vi "CSM - With Event Structure Template.vi"(5 "Init State(\"Macro: Initialize\")":string="Macro: Initialize", 7 "Name(\"\" to use uuid)":string="Event CSM") -> ()   [LabVIEW 2014]
doc: "Template for building CSM Module with User Interface. Event Structure is included in template for processing user operations.\n\n<b>Inputs:</b>\n - <b>Name(\"\" to use uuid)</b>: Module Name\n - If Input is \"\", an uuid will be used for module name. The module is marked as stand-alone mode and will not be included in module list.\n - Fi Input end with '#', the module will worked in worker mode. Modules with the same name will shared the same message queue. Any external message will be processed by one of the modules, depending who is free.\n - Otherwise, the input string will be used as module name, which should be unique in system. CSM will go to \"Critical Error\" state if duplicated module name is used in system.\n\n<b>Outputs:</b>\n - N/A"
uses:
  _Support/Priority Queue/Priority Queue.lvclass/Priority Queue.ctl
  AdvanceAPI/CSM - Revert Arguments-Safe String.vi
  _Support/Common/Trim Single line Text.vi
  _Support/Process/CSMP-Async Call.vi
  _Support/GlobalEvent/GEvt-Generate Status Log.vi
  _Support/Process/CSMP-Broadcast.vi
  _Support/GlobalEvent/GEvt-Generate Interrupt Log.vi
  _Support/GlobalEvent/GEvt-Generate Register Log.vi
  _Support/Process/CSMP-Register Status.vi
  _Support/GlobalEvent/GEvt-Generate Unregister Log.vi
  _Support/Process/CSMP-Unregister Status.vi
  _Support/Process/CSMP-Sync Call.vi
  _Support/CSMQ/_CSMObj-Unlock.vi
  _Support/Process/CSMP-PostPostMsg.vi
  _Support/Process/CSMP-PostSendMsg.vi
  _Support/CSMQ/_CSMObj-Lock State.vi
  _Support/Common/Splite Reason String Part.vi
  _Support/CSMQ/_CSMOFGV Release.vi
  _Support/Common/Remove Comments from Line.vi
  _Support/Common/Splite Single-line Message.vi
  _Support/Common/Parse Next Single-line State.vi
  _Support/CSMQ/_CSMOFGV Dequeue.vi
  _Support/CSMQ/_CSMObj-Log Error if in a Remote Session.vi
  _Support/GlobalEvent/GEvt-Generate State Change Log.vi
  _Support/GlobalEvent/GEvt-Generate Remaining States Log.vi
  _Support/GlobalEvent/GEvt-Generate Complete Log.vi
  AdvanceAPI/CSM - Keywords.vi
  _Support/CSMQ/_CSMObj-Message Check.vi
  _Support/CSMQ/_CSMObj-Enqueue Cross-Module Message.vi
  _Support/CSMQ/_CSMOFGV Get.vi
  _Support/FGV-BroadcastRegistry/Cache-Broadcast Registry Search Result.vi
  AdvanceAPI/CSM - Register Status Change.vi
  AdvanceAPI/CSM - Unregister Status Change.vi
  _Support/Common/Hex Str to U8 Data.vi
  _Support/Common/Concatenate State with Arguments.vi
  _Support/Common/U8 Data to Hex Str.vi
  Build State String with Arguments++.vi
  _Support/Priority Queue/Dequeue Element.vi
  _Support/Priority Queue/Enqueue Element.vi
  Utility/Trim Both Whitespace.vi
  _Support/CSMQ/_CSMOFGV.vi
  Utility/Build Error Cluster.vi
  _Support/FGV-BroadcastRegistry/FGV-BroadcastRegistry.vi
  _Support/FGV-BroadcastRegistry/global-Broadcast Cache Change Flag.vi
  _Support/GlobalEvent/FGV-StatusChangeEventRef.vi
  _Support/CSMQ/_CSMOFGV Obtain.vi
  _Support/GlobalEvent/FGV-GlobalEventRef.vi
  Communicable State Machine.lvlib
panel:
  out "State History":string
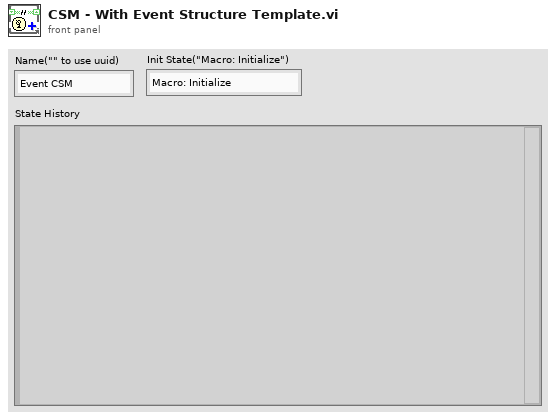
[diagram p1: front panel]
types:
  T1 = enum32{"Invalid", "Standard", "Closed", "Hidden", "Minimized", "Maximized"}
  T2 = enum32{"invalid app kind", "Development System", "Run Time System", "Student Edition", "Embedded LabVIEW", "Evaluation", "Custom"}
  T3 = typedef "Communicable State Machine.lvlib/_CSM_Response Source Message.ctl" = cluster{"‘State":string, "’Arguments":string, "’Error":errorcluster}
  T4 = cluster{"Core":cluster{"Current VI Reference":refnum<vi>, "Close Panel on Exit?":bool}, "Your Boolean data":bool, "Your string data":string}
  T5 = cluster{"Current VI Reference":refnum<vi>, "Close Panel on Exit?":bool}
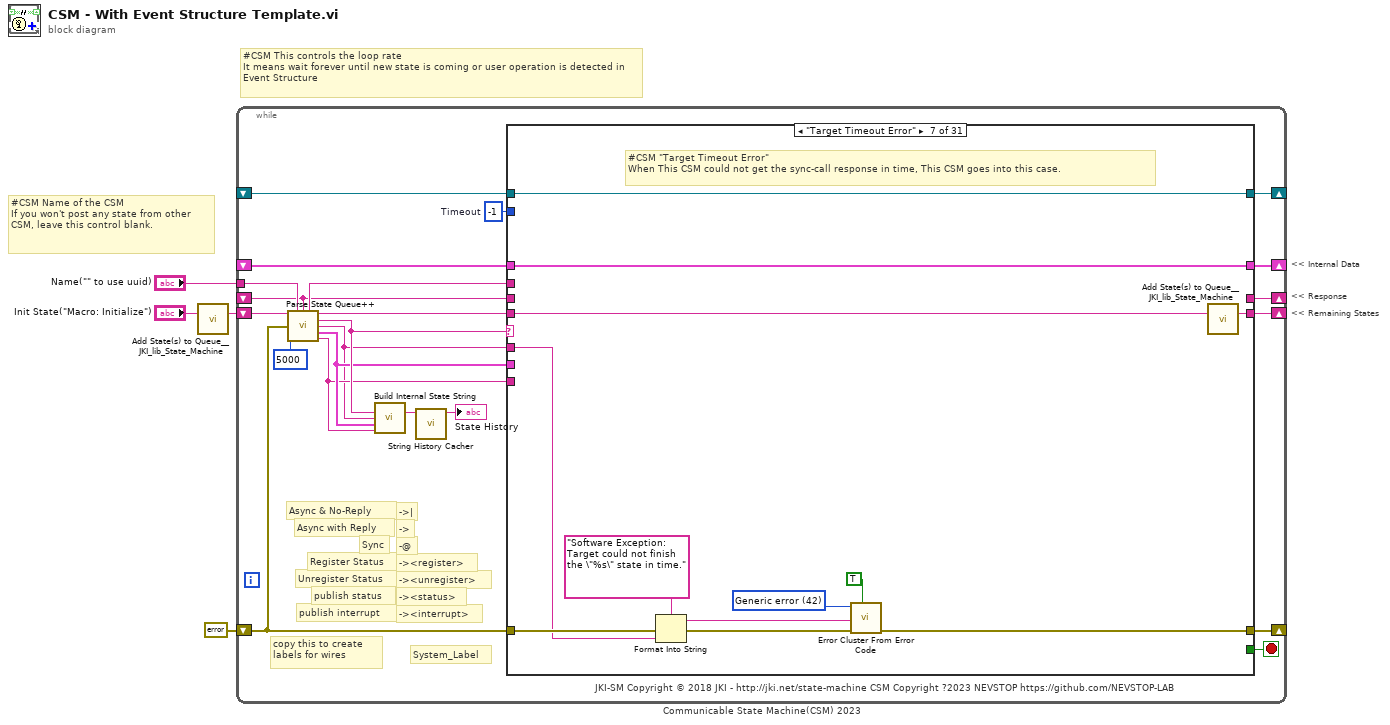
[diagram p0: block diagram]
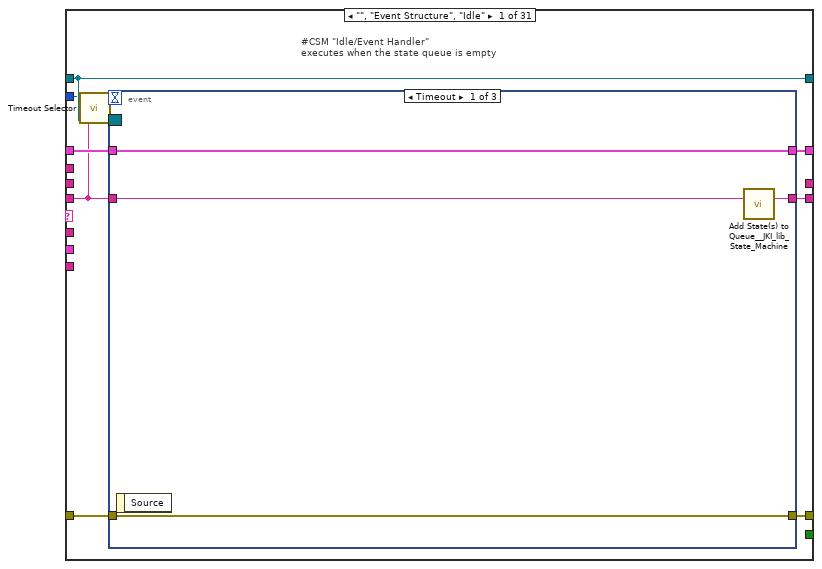
[diagram p2: hidden frame]
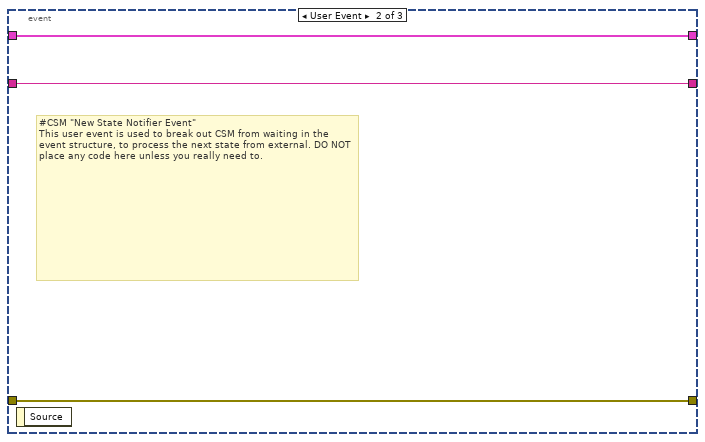
[diagram p3: hidden frame]
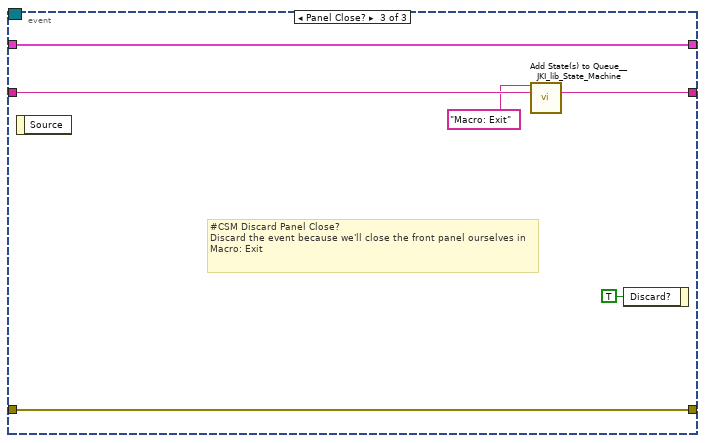
[diagram p4: hidden frame]
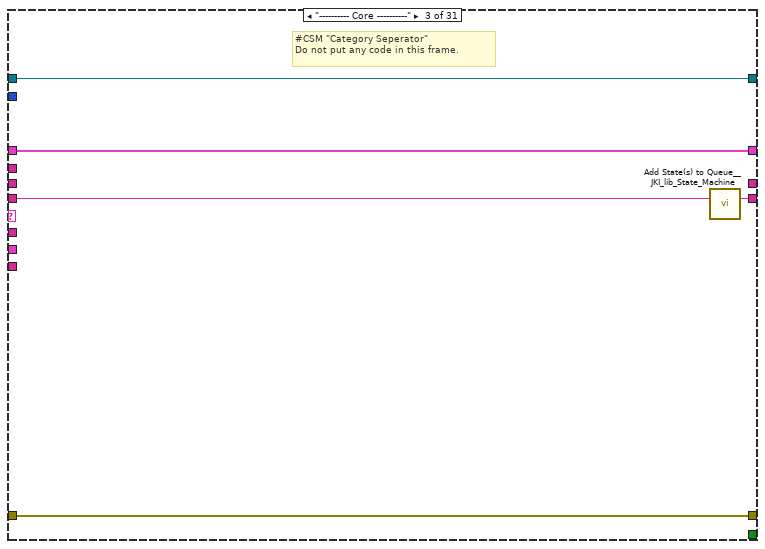
[diagram p6: hidden frame]
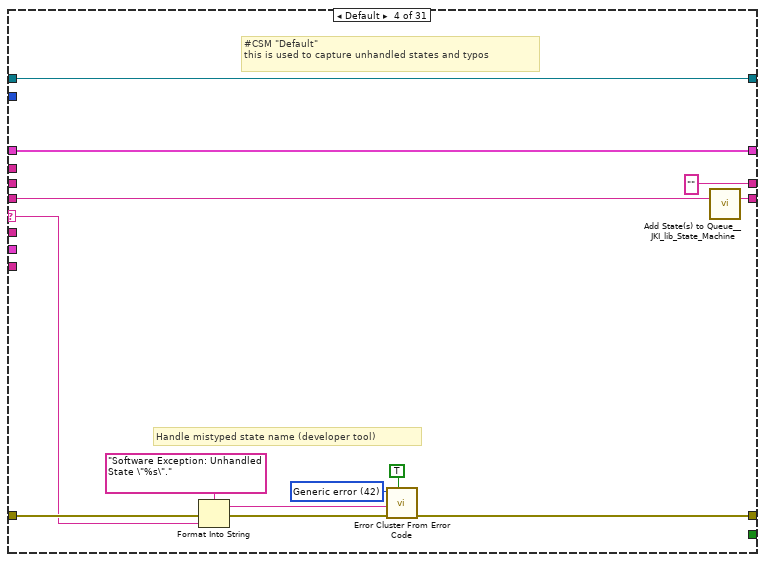
[diagram p7: hidden frame]
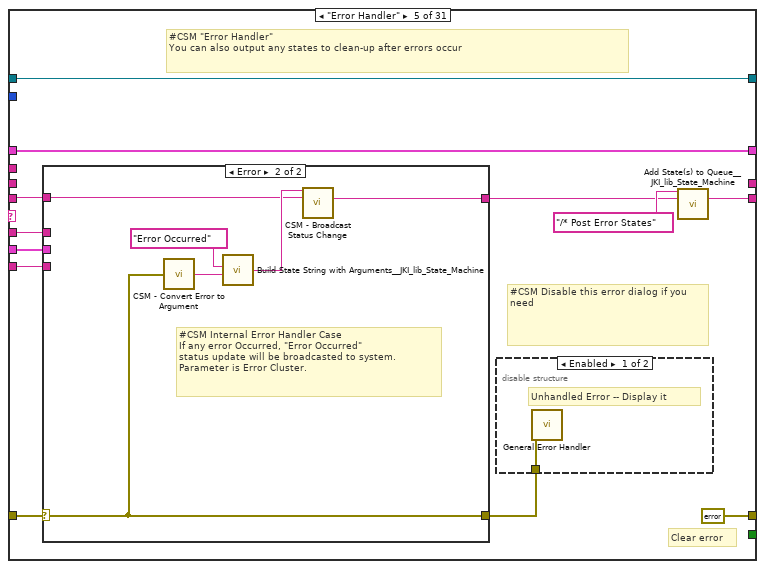
[diagram p8: hidden frame]
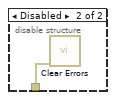
[diagram p9: hidden frame]
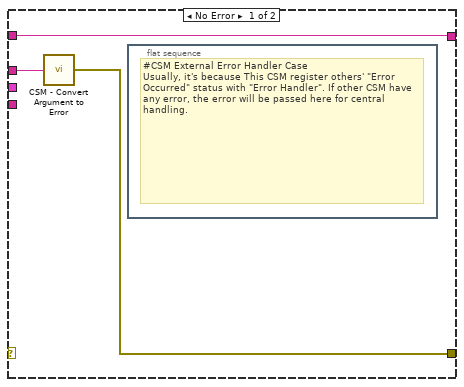
[diagram p10: hidden frame]
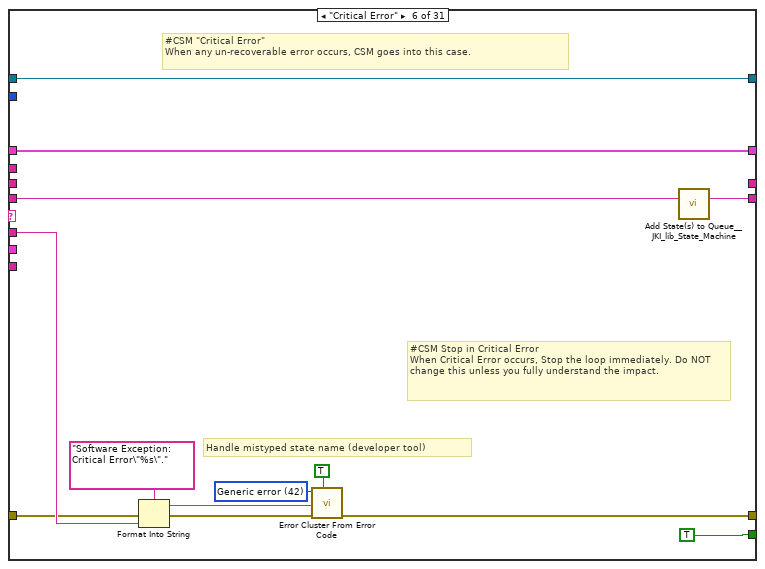
[diagram p11: hidden frame]
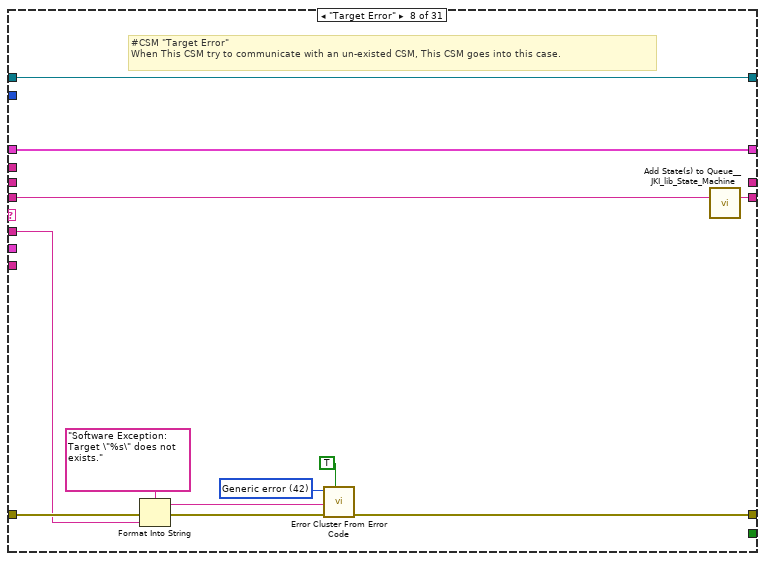
[diagram p12: hidden frame]
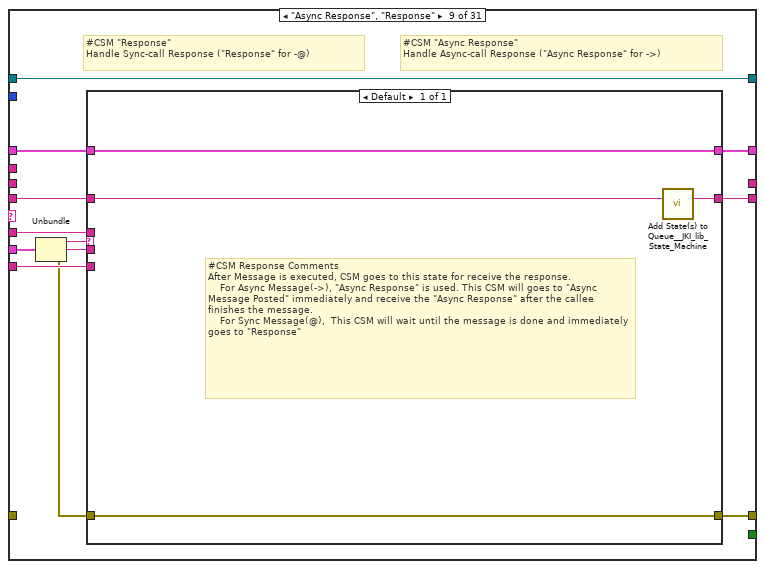
[diagram p13: hidden frame]
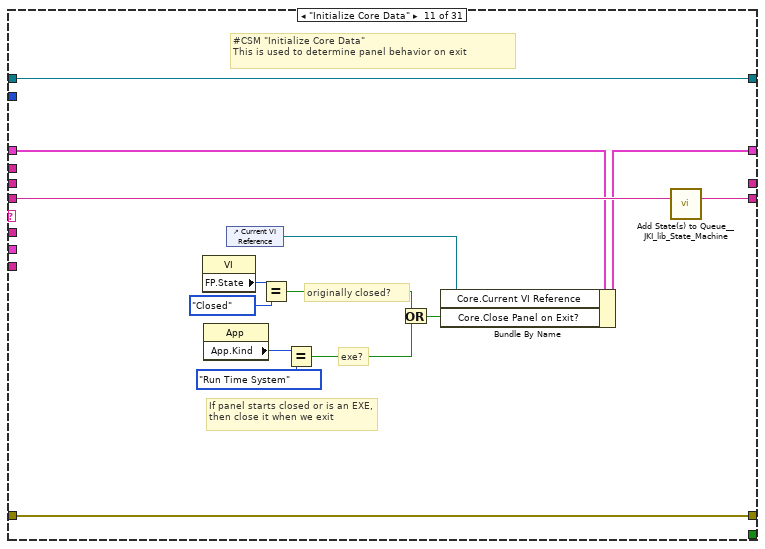
[diagram p15: hidden frame]
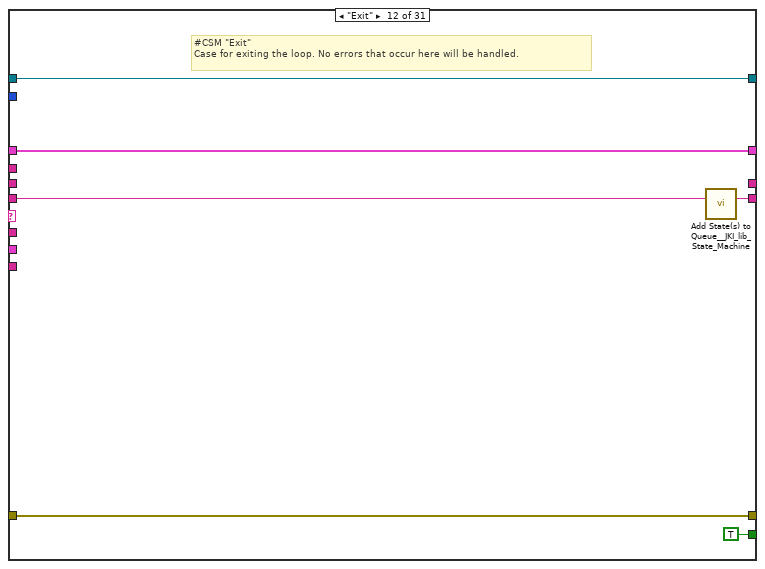
[diagram p16: hidden frame]
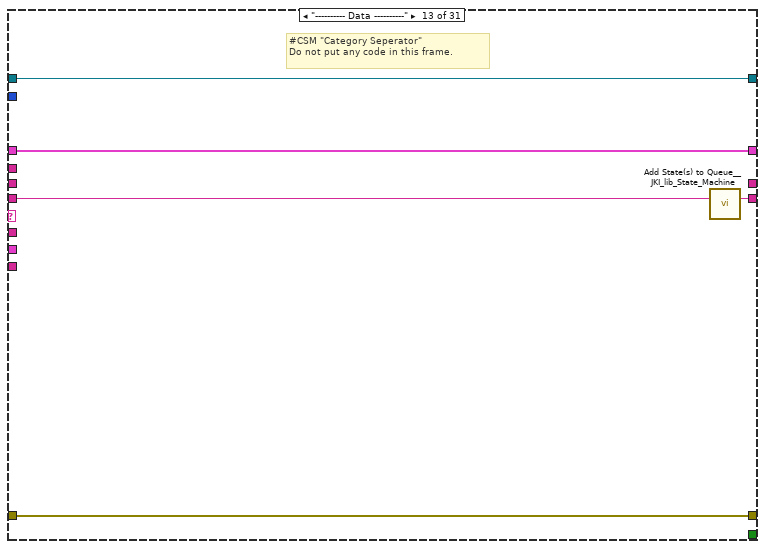
[diagram p17: hidden frame]
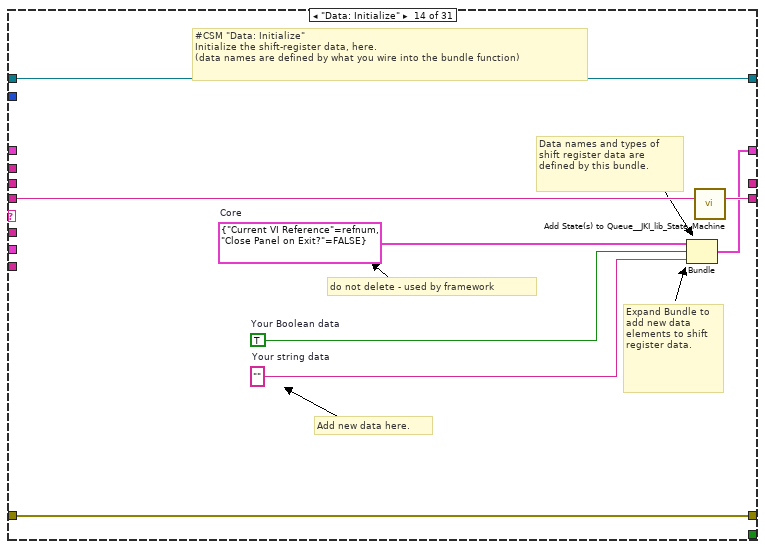
[diagram p18: hidden frame]
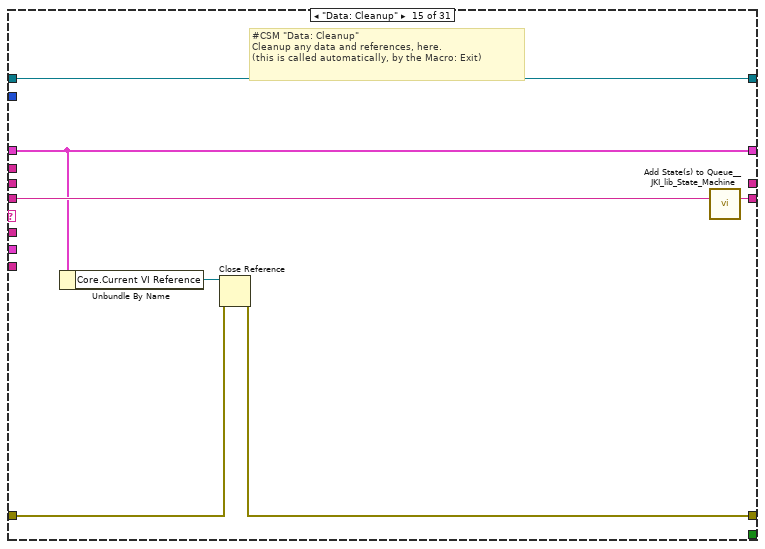
[diagram p19: hidden frame]
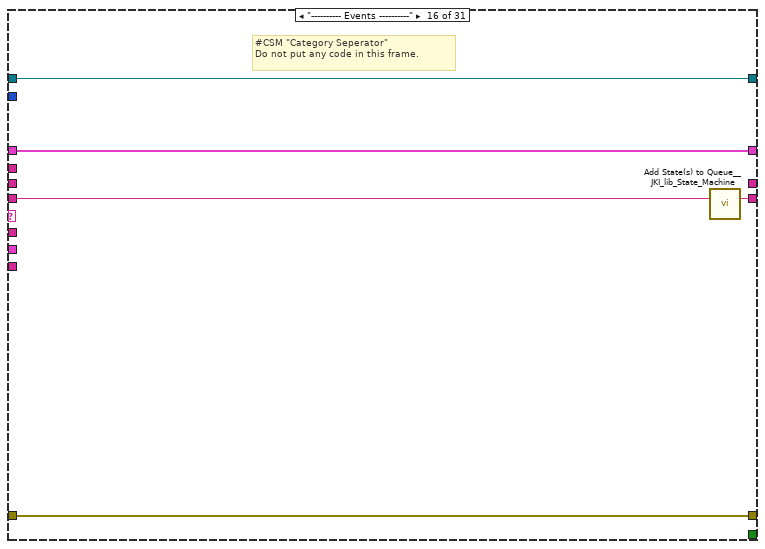
[diagram p20: hidden frame]
diagram:
  # "<< Internal Data"
  # "<< Response"
  # "<< Remaining States"
  # "#CSM Name of the CSM\nIf you won't post any state from other CSM, leave this control blank."
  # "#CSM This controls the loop rate\nIt means wait forever until new state is coming or user operation is detected in Event Structure"
  n1 = call <vilib>:"Add State(s) to Queue__JKI_lib_State_Machine.vi"("State(s) in (\"\")"="Init State(\"Macro: Initialize\")") -> ("States Out"=w4:string)  [unwired: 14 in]
  n2 = while "Communicable State Machine(CSM) 2023" {
    shift-right: [w21] -> _
    shift-left: _ -> [w20]
    shift-right: [w24] -> _
    shift-left: errorcluster {"status"=FALSE, "code"=0, "source"=""} ("error out") -> [w18]
    shift-right: [w23] -> _
    shift-left: w4 -> [w25]
    tunnel: "Name(\"\" to use uuid)" -> [w13]
    shift-right: [w16] -> _
    shift-left: _ -> [w6]
    shift-right: [w15] -> _
    shift-left: _ -> [w14]
    stop <- w22 stop-if-true
    w19 = -1  # Timeout
    # "-><interrupt>"
    # "-><status>"
    # "-><unregister>"
    # "-><register>"
    # "-@"
    # "->"
    # "->|"
    # "publish interrupt"
    # "publish status"
    # "Unregister Status"
    # "Register Status"
    # "Sync"
    # "Async with Reply"
    # "Async & No-Reply"
    # "copy this to create labels for wires"
    # "System_Label"
    # "JKI-SM Copyright © 2018 JKI - http://jki.net/state-machine CSM Copyright ?2023 NEVSTOP https://github.com/NEVSTOP-LAB"
    n3 = call "Parse State Queue++.vi"("State Queue"=w25, "Name(\"\" to use uuid)"=w13, "Response Arguments"=w6, "Error In (no error)"=w18, "Response Timeout(5000ms)"=5000 ("Response Timeout(1000ms)")) -> ("Name Used"=w7:string, "Remaining States"=w26:string, "Current State"=w10:string, "Arguments"=w5:string, ">> Response Source Message >>"=w9:T3, ">> Source CSM >>"=w8:string)  [unwired: 5 in]
    n4 = call "Build Internal State String.vi"("State"=w10, "Arguments (\"\")"=w5, ">> Response Source Message >>"=w9, "Source (\"\")"=w8) -> ("State with Arguments"=w11:string)  [unwired: 11 in]
    n5 = call "String History Cacher.vi"("String"=w11) -> ("String Cache"=→"State History":string)  [unwired: 10 in]
    n6 = case shown="\"Target Timeout Error\"" w10 {
      selector: w10 -> [_ _ _ w60 _ _ _ _ _ _ _ _ _ _ _ _ _ _ _ _ _ _ _ _ _ _ _ _ _ _ _]
      tunnel: w26 -> [w27 w52 w57 w64 w75 w105 w113 w125 w140 w149 w164 w170 w175 w183 w190 w195 w202 w206 w212 w217 w224 w240 w310 w316 w328 w331 w336 w340 w346 w351 w356]
      tunnel: w5 -> [_ _ _ _ w73 w98 w109 w121 w134 _ _ _ _ _ _ _ _ _ _ _ w219 w234 _ _ _ _ _ _ _ _ _]
      tunnel: w20 -> [w34 w51 w54 w62 w81 w106 w111 w123 w138 w148 w157 w168 w172 _ w185 w192 w201 w205 w209 w215 w222 w236 w307 w313 w325 w330 w335 w339 w343 w348 w353]
      tunnel: [w33 w50 w55 w66 errorcluster {"status"=FALSE, "code"=0, "source"=""} ("error out") w94 w107 w119 w137 w150 w161 w167 w173 w180 w186 w193 w196 w204 w210 w214 w220 w237 w308 w314 w326 w332 w337 w341 w344 w349 w354] -> w24
      tunnel: w18 -> [w32 w50 w55 w65 w79 w95 w114 w126 _ w150 w161 w167 w173 w180 w187 w193 _ w207 w210 w214 w221 w238 w308 w314 w326 w332 w337 w341 w344 w349 w354]
      tunnel: [w35 w52 w56 w63 w77 w104 w112 w124 w141 w149 w163 w169 w174 w182 w189 w194 w202 w206 w211 w216 w223 w239 w309 w315 w327 w331 w336 w340 w345 w350 w355] -> w23
      tunnel: [_ _ _ _ _ TRUE _ _ _ _ _ TRUE _ _ _ _ _ _ _ _ _ _ _ _ _ _ _ _ _ _ _] -> w22
      tunnel: [w31 w51 w54 w62 w81 w106 w111 w123 w139 w148 w162 w168 w172 w181 w185 w192 w201 w205 w209 w215 w222 w236 w307 w313 w325 w330 w335 w339 w343 w348 w353] -> w21
      tunnel: w19 -> [w29 _ _ _ _ _ _ _ _ _ _ _ _ _ _ _ _ _ _ _ _ _ _ _ _ _ _ _ _ _ _]
      tunnel: w8 -> [_ _ _ _ w72 _ _ _ w135 _ _ _ _ _ _ _ _ _ _ _ _ _ _ _ _ _ _ _ _ _ _]
      tunnel: w9 -> [_ _ _ _ w71 _ _ _ w136 _ _ _ _ _ _ _ _ _ _ _ _ _ _ _ _ _ _ _ _ _ _]
      tunnel: [_ _ _ "" _ _ _ _ _ _ _ _ _ _ _ _ _ _ _ _ _ _ _ _ _ _ "API1 Response" _ _ _ _] -> w16
      tunnel: [w30 w49 w53 w58 w80 w96 w108 w120 w142 w147 w151 w165 w171 w176 w184 w191 w200 w203 w208 w213 w218 w233 w306 w311 w318 w329 w334 w338 w342 w347 w352] -> w15
      tunnel: w14 -> [w30 w49 w53 w58 w80 w96 w108 w120 w142 w147 w151 w165 w171 w176 w184 w191 _ w203 w208 w213 w218 w233 w306 w311 w318 w329 w334 w338 w342 w347 w352]
      tunnel: w7 -> [_ _ _ _ _ _ _ _ _ _ _ _ _ _ _ _ w199 _ _ _ _ _ _ _ _ _ _ _ _ _ _]
      tunnel: w6 -> [_ _ _ _ _ _ _ _ _ _ _ _ _ _ _ _ _ _ _ _ _ _ _ _ _ _ _ _ _ _ _]
      frame "", "Event Structure", "Idle" {
        # "#CSM \"Idle/Event Handler\"\nexecutes when the state queue is empty"
        n7 = call "Timeout Selector.vi"("Remaining States"=w27, "Timeout Expected"=w29) -> ("Timeout"=w28:i32)  [unwired: 5 in]
        n8 = event shown="[0] Timeout" {
          selector: w30 -> [_ _ _]
          dyn-events: _ -> [_ _ _]
          timeout: w28 -> [_ _ _]
          tunnel: w27 -> [w39 w41 w48]
          tunnel: [w38 w41 w47] -> w35
          tunnel: w34 -> [w36 w42 w45]
          tunnel: [w37 w40 w46] -> w33
          tunnel: w32 -> [w37 w40 w46]
          tunnel: [w36 w42 w45] -> w31
          event Timeout {
            n9 = event-data() -> ()  [unwired: 1 in, 1 out]
            n10 = call <vilib>:"Add State(s) to Queue__JKI_lib_State_Machine.vi"("State(s) in (\"\")"=w39) -> ("States Out"=w38:string)  [unwired: 14 in]
          }
          event User Event {
            # "#CSM \"New State Notifier Event\"\nThis user event is used to break out CSM from waiting in the event structure, to process the next state from external. DO NOT place any code here unless you really need to."
            n11 = event-data() -> ()  [unwired: 1 in, 1 out]
          }
          event Panel Close? {
            # "#CSM Discard Panel Close?\nDiscard the event because we'll close the front panel ourselves in Macro: Exit"
            n12 = event-data() -> ()  [unwired: 1 in, 1 out]
            n13 = call <vilib>:"Add State(s) to Queue__JKI_lib_State_Machine.vi"("State(s) in Front (\"\")"="Macro: Exit", "State(s) in (\"\")"=w48) -> ("States Out"=w47:string)  [unwired: 13 in]
            n14 = event-data("Discard?"=TRUE) -> ()  [unwired: 1 in, 1 out]
          }
        }
      }
      frame "CSM Documentation" {
        # "#CSM \"Documentation\"\nCase for holding CSM Documenation"
        # "CSM Documentation"
        # "#CSM Commenting\nTo add a comment use \"//\" or \"#\" and all text to the right will be ignored\n\nCommenting Example:\nUI: Initialize // This initializes the UI\n// Another comment line"
        # "#CSM State Syntax\n\n    // Local Message Example\n    DoSth: DoA >> Arguments\n\n    // Sync Call Example\n    API: xxxx >> Arguments -@ TargetModule\n\n    // Async Call Example\n    API: xxxx >> Arguments -> TargetModule\n\n    // Async Call without Reply Example\n    API: xxxx >> Arguments ->| TargetModule\n\n    // Broadcast normal status:\n    Status >> StatusArguments  -><status>\n\n    // Broadcast Interrupt status:\n    Interrupt >> StatusArguments  -><interrupt>\n\n    // Register Source Module's status to Handler Module\n    Status@Source Module >> Handler Module@Handler Module -><register>\n\n    // Unegister Source Module's status\n    Status@Source Module >> Handler Module -><unregister>"
        # "#CSM README FIRST\n\nCSM is a LabVIEW application framework that builds upon JKI State Machine (CSM). It follows the pattern of CSM and extends the keywords to describe message communication between CSM modules, including concepts such as Sync-Message, Async-Message, Subscription/Unsubscription of status - essential elements for creating reusable code modules. For more information, please visit the CSM wiki: https://github.com/NEVSTOP-LAB/JKI-State-Machine-Plus-Plus/wiki\n\nFor instructions on JKI State Machine, visit: \n    http://jki.net/state-machine/\nFor information about CSM, visit: \n    https://github.com/NEVSTOP-LAB"
      }
      frame "---------- Core ----------" {
        # "#CSM \"Category Seperator\"\nDo not put any code in this frame."
        n15 = call <vilib>:"Add State(s) to Queue__JKI_lib_State_Machine.vi"("State(s) in (\"\")"=w57) -> ("States Out"=w56:string)  [unwired: 14 in]
      }
      frame Default {
        w69 = 42 items=["No error", "Argument error", "Memory is full", "Out of zone", "End of file", "File already open", "Generic file I/O error", "File not found", "File permission error", "Disk is full", "Duplicate path", "Too many files open", "System feature not enabled", "Resource file not found", "Cannot add resource", "Resource not found", "Image not found", "Image memory error", "Pen does not exist", "Config type invalid", "Config token not found", "Config parse error", "Config memory error", "Bad external code format", "Bad external code offset", "External code not present", "Null window", "Destroy window error", "Null menu", "Print aborted", "Bad print record", "Print driver error", "Windows error during printing", "Memory error during printing", "Print dialog error", "Generic print error", "Invalid device refnum", "Device not found", "Device parameter error", "Device unit error", "Cannot open device", "Device call aborted", "Generic error", "Cancelled by user", "Object ID too low", "Object ID too high", "Object not in heap", "Unknown heap", "Unknown object (invalid DefProc)", "Unknown object (DefProc not in table)", "Message out of range", "Invalid (null) method", "Unknown message", "Manager call not supported", "Bad address", "Network operation in progress", "Network operation timed out", "Connection is busy", "Network attribute not supported", "Network error", "Address in use", "System out of memory", "Connection aborted", "Connection refused", "Not connected", "Already connected", "Connection closed", "Initialization error (interapplication manager)", "Bad occurrence", "Wait on unbound occurrence handler", "Occurrence queue overflow", "Datalog type conflict", "Unused", "Unrecognized type (interapplication manager)", "Memory corrupt", "Failed to make temporary DLL", "Old CIN version", "Drag socket not found", "Failed to load drop-object", "Failed to register OLE object", "Failed to release OLE object", "Format specifier type mismatch", "Unknown format specifier", "Too few format specifiers", "Too many format specifiers", "Scan failed", "Newer CIN version", "Error converting to variant", "Runtime menu error", "Password tampered", "Variant attribute not found", "Incompatible variant data type", "Event data is not available", "Event Store is not present", "Occurrence is not found", "Event Queue is not created", "Event info is not available", "Refnum passed is NULL", "Error retrieving Class GUID", "Error retrieving CoClass GUID", "Error retrieving TypeLib GUID.", "Bad built application magic bytes.", "Specific driver is different from the specific driver associated with the Logical Name.", "There is no session opened to the class driver.", "Max Error", "MAX - Error with config objects", "MAX - Error loading configuration", "MAX - Group not supported"]
        # "#CSM \"Default\"\nthis is used to capture unhandled states and typos"
        # "Handle mistyped state name (developer tool)"
        n16 = Format Into String(format string="Software Exception: Unhandled State \"%s\"." ("message"), error in=w65, w60) -> (resulting string=w68:string, error out=w67:errorcluster)  [unwired: 1 in]
        n17 = call <vilib>:"Error Cluster From Error Code.vi"("show call chain? (False)"=TRUE, "error in (no error)"=w67, "error message (\"\")"=w68, "error code (0)"=w69) -> ("error out"=w66:errorcluster)  [unwired: 5 in]
        n18 = call <vilib>:"Add State(s) to Queue__JKI_lib_State_Machine.vi"("State(s) in (\"\")"=w64) -> ("States Out"=w63:string)  [unwired: 14 in]
      }
      frame "Error Handler" {
        # "#CSM Disable this error dialog if you need"
        # "#CSM \"Error Handler\"\nYou can also output any states to clean-up after errors occur"
        # "Clear error"
        n19 = case shown="Error" w79 {
          selector: w79 -> [_ w88]
          tunnel: [w86 w90] -> w76
          tunnel: w75 -> [w86 w89]
          tunnel: [w85 w88] -> w74
          tunnel: w73 -> [w87 _]
          tunnel: w72 -> [_ _]
          tunnel: w71 -> [_ _]
          frame No Error {
            n20 = call "CSM - Convert Argument to Error.vi"("Argument"=w87) -> ("error"=w85:errorcluster)  [unwired: 4 in]
            n21 = flat-sequence {
              frame #0 {
                # "#CSM External Error Handler Case\nUsually, it's because This CSM register others' \"Error Occurred\" status with \"Error Handler\". If other CSM have any error, the error will be passed here for central handling."
              }
            }
          }
          frame Error {
            # "#CSM Internal Error Handler Case \nIf any error Occurred, \"Error Occurred\" \nstatus update will be broadcasted to system.\nParameter is Error Cluster."
            n22 = call "CSM - Convert Error to Argument.vi"("error in (no error)"=w88) -> ("Arguments"=w92:string)  [unwired: 4 in]
            n23 = call <vilib>:"Build State String with Arguments__JKI_lib_State_Machine.vi"("Arguments (\"\")"=w92, "State"="Error Occurred" ("Status with Arguments")) -> ("State with Arguments"=w91:string)  [unwired: 4 in]
            n24 = call "CSM - Broadcast Status Change.vi"("Status with Arguments"=w91, "State Queue"=w89) -> ("Remaining States"=w90:string)  [unwired: 13 in]
          }
        }
        n25 = disable-structure shown="Enabled" {
          disable-tunnel: w74 -> [w83 w84]
          frame Enabled {
            # "Unhandled Error -- Display it"
            n26 = call <vilib>:"General Error Handler.vi"("error in (no error)"=w83) -> ()  [unwired: 10 in, 5 out]
          }
          frame Disabled {
            n27 = call <vilib>:"Clear Errors.vi"("error in (no error)"=w84) -> ()  [unwired: 5 in, 2 out]
          }
        }
        n28 = call <vilib>:"Add State(s) to Queue__JKI_lib_State_Machine.vi"("State(s) in Front (\"\")"="/* Post Error States", "State(s) in (\"\")"=w76) -> ("States Out"=w77:string)  [unwired: 13 in]
      }
      frame "Critical Error" {
        w102 = 42 items=["No error", "Argument error", "Memory is full", "Out of zone", "End of file", "File already open", "Generic file I/O error", "File not found", "File permission error", "Disk is full", "Duplicate path", "Too many files open", "System feature not enabled", "Resource file not found", "Cannot add resource", "Resource not found", "Image not found", "Image memory error", "Pen does not exist", "Config type invalid", "Config token not found", "Config parse error", "Config memory error", "Bad external code format", "Bad external code offset", "External code not present", "Null window", "Destroy window error", "Null menu", "Print aborted", "Bad print record", "Print driver error", "Windows error during printing", "Memory error during printing", "Print dialog error", "Generic print error", "Invalid device refnum", "Device not found", "Device parameter error", "Device unit error", "Cannot open device", "Device call aborted", "Generic error", "Cancelled by user", "Object ID too low", "Object ID too high", "Object not in heap", "Unknown heap", "Unknown object (invalid DefProc)", "Unknown object (DefProc not in table)", "Message out of range", "Invalid (null) method", "Unknown message", "Manager call not supported", "Bad address", "Network operation in progress", "Network operation timed out", "Connection is busy", "Network attribute not supported", "Network error", "Address in use", "System out of memory", "Connection aborted", "Connection refused", "Not connected", "Already connected", "Connection closed", "Initialization error (interapplication manager)", "Bad occurrence", "Wait on unbound occurrence handler", "Occurrence queue overflow", "Datalog type conflict", "Unused", "Unrecognized type (interapplication manager)", "Memory corrupt", "Failed to make temporary DLL", "Old CIN version", "Drag socket not found", "Failed to load drop-object", "Failed to register OLE object", "Failed to release OLE object", "Format specifier type mismatch", "Unknown format specifier", "Too few format specifiers", "Too many format specifiers", "Scan failed", "Newer CIN version", "Error converting to variant", "Runtime menu error", "Password tampered", "Variant attribute not found", "Incompatible variant data type", "Event data is not available", "Event Store is not present", "Occurrence is not found", "Event Queue is not created", "Event info is not available", "Refnum passed is NULL", "Error retrieving Class GUID", "Error retrieving CoClass GUID", "Error retrieving TypeLib GUID.", "Bad built application magic bytes.", "Specific driver is different from the specific driver associated with the Logical Name.", "There is no session opened to the class driver.", "Max Error", "MAX - Error with config objects", "MAX - Error loading configuration", "MAX - Group not supported"]
        # "#CSM \"Critical Error\"\nWhen any un-recoverable error occurs, CSM goes into this case."
        # "#CSM Stop in Critical Error\nWhen Critical Error occurs, Stop the loop immediately. Do NOT change this unless you fully understand the impact."
        # "Handle mistyped state name (developer tool)"
        n29 = Format Into String(format string="Software Exception: Critical Error\"%s\"." ("message"), error in=w95, w98) -> (resulting string=w101:string, error out=w100:errorcluster)  [unwired: 1 in]
        n30 = call <vilib>:"Error Cluster From Error Code.vi"("show call chain? (False)"=TRUE, "error in (no error)"=w100, "error message (\"\")"=w101, "error code (0)"=w102) -> ("error out"=w94:errorcluster)  [unwired: 5 in]
        n31 = call <vilib>:"Add State(s) to Queue__JKI_lib_State_Machine.vi"("State(s) in (\"\")"=w105) -> ("States Out"=w104:string)  [unwired: 14 in]
      }
      frame "Target Timeout Error" {
        w117 = 42 items=["No error", "Argument error", "Memory is full", "Out of zone", "End of file", "File already open", "Generic file I/O error", "File not found", "File permission error", "Disk is full", "Duplicate path", "Too many files open", "System feature not enabled", "Resource file not found", "Cannot add resource", "Resource not found", "Image not found", "Image memory error", "Pen does not exist", "Config type invalid", "Config token not found", "Config parse error", "Config memory error", "Bad external code format", "Bad external code offset", "External code not present", "Null window", "Destroy window error", "Null menu", "Print aborted", "Bad print record", "Print driver error", "Windows error during printing", "Memory error during printing", "Print dialog error", "Generic print error", "Invalid device refnum", "Device not found", "Device parameter error", "Device unit error", "Cannot open device", "Device call aborted", "Generic error", "Cancelled by user", "Object ID too low", "Object ID too high", "Object not in heap", "Unknown heap", "Unknown object (invalid DefProc)", "Unknown object (DefProc not in table)", "Message out of range", "Invalid (null) method", "Unknown message", "Manager call not supported", "Bad address", "Network operation in progress", "Network operation timed out", "Connection is busy", "Network attribute not supported", "Network error", "Address in use", "System out of memory", "Connection aborted", "Connection refused", "Not connected", "Already connected", "Connection closed", "Initialization error (interapplication manager)", "Bad occurrence", "Wait on unbound occurrence handler", "Occurrence queue overflow", "Datalog type conflict", "Unused", "Unrecognized type (interapplication manager)", "Memory corrupt", "Failed to make temporary DLL", "Old CIN version", "Drag socket not found", "Failed to load drop-object", "Failed to register OLE object", "Failed to release OLE object", "Format specifier type mismatch", "Unknown format specifier", "Too few format specifiers", "Too many format specifiers", "Scan failed", "Newer CIN version", "Error converting to variant", "Runtime menu error", "Password tampered", "Variant attribute not found", "Incompatible variant data type", "Event data is not available", "Event Store is not present", "Occurrence is not found", "Event Queue is not created", "Event info is not available", "Refnum passed is NULL", "Error retrieving Class GUID", "Error retrieving CoClass GUID", "Error retrieving TypeLib GUID.", "Bad built application magic bytes.", "Specific driver is different from the specific driver associated with the Logical Name.", "There is no session opened to the class driver.", "Max Error", "MAX - Error with config objects", "MAX - Error loading configuration", "MAX - Group not supported"]
        # "#CSM \"Target Timeout Error\"\nWhen This CSM could not get the sync-call response in time, This CSM goes into this case."
        n32 = Format Into String(format string="Software Exception: Target could not finish the \"%s\" state in time." ("message"), error in=w114, w109) -> (resulting string=w116:string, error out=w115:errorcluster)  [unwired: 1 in]
        n33 = call <vilib>:"Error Cluster From Error Code.vi"("show call chain? (False)"=TRUE, "error in (no error)"=w115, "error message (\"\")"=w116, "error code (0)"=w117) -> ("error out"=w107:errorcluster)  [unwired: 5 in]
        n34 = call <vilib>:"Add State(s) to Queue__JKI_lib_State_Machine.vi"("State(s) in (\"\")"=w113) -> ("States Out"=w112:string)  [unwired: 14 in]
      }
      frame "Target Error" {
        w129 = 42 items=["No error", "Argument error", "Memory is full", "Out of zone", "End of file", "File already open", "Generic file I/O error", "File not found", "File permission error", "Disk is full", "Duplicate path", "Too many files open", "System feature not enabled", "Resource file not found", "Cannot add resource", "Resource not found", "Image not found", "Image memory error", "Pen does not exist", "Config type invalid", "Config token not found", "Config parse error", "Config memory error", "Bad external code format", "Bad external code offset", "External code not present", "Null window", "Destroy window error", "Null menu", "Print aborted", "Bad print record", "Print driver error", "Windows error during printing", "Memory error during printing", "Print dialog error", "Generic print error", "Invalid device refnum", "Device not found", "Device parameter error", "Device unit error", "Cannot open device", "Device call aborted", "Generic error", "Cancelled by user", "Object ID too low", "Object ID too high", "Object not in heap", "Unknown heap", "Unknown object (invalid DefProc)", "Unknown object (DefProc not in table)", "Message out of range", "Invalid (null) method", "Unknown message", "Manager call not supported", "Bad address", "Network operation in progress", "Network operation timed out", "Connection is busy", "Network attribute not supported", "Network error", "Address in use", "System out of memory", "Connection aborted", "Connection refused", "Not connected", "Already connected", "Connection closed", "Initialization error (interapplication manager)", "Bad occurrence", "Wait on unbound occurrence handler", "Occurrence queue overflow", "Datalog type conflict", "Unused", "Unrecognized type (interapplication manager)", "Memory corrupt", "Failed to make temporary DLL", "Old CIN version", "Drag socket not found", "Failed to load drop-object", "Failed to register OLE object", "Failed to release OLE object", "Format specifier type mismatch", "Unknown format specifier", "Too few format specifiers", "Too many format specifiers", "Scan failed", "Newer CIN version", "Error converting to variant", "Runtime menu error", "Password tampered", "Variant attribute not found", "Incompatible variant data type", "Event data is not available", "Event Store is not present", "Occurrence is not found", "Event Queue is not created", "Event info is not available", "Refnum passed is NULL", "Error retrieving Class GUID", "Error retrieving CoClass GUID", "Error retrieving TypeLib GUID.", "Bad built application magic bytes.", "Specific driver is different from the specific driver associated with the Logical Name.", "There is no session opened to the class driver.", "Max Error", "MAX - Error with config objects", "MAX - Error loading configuration", "MAX - Group not supported"]
        # "#CSM \"Target Error\"\nWhen This CSM try to communicate with an un-existed CSM, This CSM goes into this case."
        n35 = Format Into String(format string="Software Exception: Target \"%s\" does not exists." ("message"), error in=w126, w121) -> (resulting string=w128:string, error out=w127:errorcluster)  [unwired: 1 in]
        n36 = call <vilib>:"Error Cluster From Error Code.vi"("show call chain? (False)"=TRUE, "error in (no error)"=w127, "error message (\"\")"=w128, "error code (0)"=w129) -> ("error out"=w119:errorcluster)  [unwired: 5 in]
        n37 = call <vilib>:"Add State(s) to Queue__JKI_lib_State_Machine.vi"("State(s) in (\"\")"=w125) -> ("States Out"=w124:string)  [unwired: 14 in]
      }
      frame "Async Response", "Response" {
        # "#CSM \"Async Response\"\nHandle Async-call Response (\"Async Response\" for ->)"
        # "#CSM \"Response\"\nHandle Sync-call Response (\"Response\" for -@)"
        n38 = Unbundle(w136) -> ("‘State"=w133:string, "’Arguments"=w132:string, "’Error"=w131:errorcluster)
        n39 = case shown="Default" w133 {
          tunnel: [w143] -> w141
          tunnel: w140 -> [w144]
          tunnel: [w146] -> w139
          tunnel: w138 -> [w146]
          tunnel: [w145] -> w137
          tunnel: w131 -> [w145]
          tunnel: w135 -> [_]
          tunnel: w134 -> [_]
          tunnel: w132 -> [_]
          frame Default {
            # "#CSM Response Comments\nAfter Message is executed, CSM goes to this state for receive the response.\n    For Async Message(->), \"Async Response\" is used. This CSM will goes to \"Async Message Posted\" immediately and receive the \"Async Response\" after the callee finishes the message.\n    For Sync Message(@),  This CSM will wait until the message is done and immediately goes to \"Response\""
            n40 = call <vilib>:"Add State(s) to Queue__JKI_lib_State_Machine.vi"("State(s) in (\"\")"=w144) -> ("States Out"=w143:string)  [unwired: 14 in]
          }
        }
      }
      frame "Async Message Posted" {
        # "#CSM \"Async Message Posted\"\nAfter Async Message is posted (-> or ->| ), CSM goes to this state for post-action.\nYou can use Argument - State to tell which Async Message is called."
      }
      frame "Initialize Core Data" {
        # "#CSM \"Initialize Core Data\"\nThis is used to determine panel behavior on exit"
        # "originally closed?"
        # "exe?"
        # "If panel starts closed or is an EXE, then close it when we exit"
        n41 = property class="VI"() -> ("FP.State"=w154:T1)  [unwired: 2 in, 2 out]
        n42 = property class="App"() -> ("App.Kind"=w160:T2)  [unwired: 2 in, 2 out]
        n43 = control-ref of="Current VI Reference"() -> (w155:refnum<vi>)
        n44 = Equal?(x=w154, y=T1."Closed" ("Front Panel Window:State")) -> (x = y?=w152:bool)
        n45 = Equal?(x=w160, y=T2."Run Time System" ("Application:Kind")) -> (x = y?=w158:bool)
        n46 = Or(x=w152, y=w158) -> (x .or. y?=w156:bool)
        n47 = Bundle By Name(cluster=w157, "Core.Current VI Reference"=w155, "Core.Close Panel on Exit?"=w156) -> (w162:T4)
        n48 = call <vilib>:"Add State(s) to Queue__JKI_lib_State_Machine.vi"("State(s) in (\"\")"=w164) -> ("States Out"=w163:string)  [unwired: 14 in]
      }
      frame "Exit" {
        # "#CSM \"Exit\"\nCase for exiting the loop. No errors that occur here will be handled."
        n49 = call <vilib>:"Add State(s) to Queue__JKI_lib_State_Machine.vi"("State(s) in (\"\")"=w170) -> ("States Out"=w169:string)  [unwired: 14 in]
      }
      frame "---------- Data ----------" {
        # "#CSM \"Category Seperator\"\nDo not put any code in this frame."
        n50 = call <vilib>:"Add State(s) to Queue__JKI_lib_State_Machine.vi"("State(s) in (\"\")"=w175) -> ("States Out"=w174:string)  [unwired: 14 in]
      }
      frame "Data: Initialize" {
        w177 = T5 {"Current VI Reference"=refnum, "Close Panel on Exit?"=FALSE}  # Core
        w179 = TRUE  # Your Boolean data
        w178 = ""  # Your string data
        # "do not delete - used by framework"
        # "Expand Bundle to add new data elements to shift register data."
        # "Add new data here."
        # "Data names and types of shift register data are defined by this bundle."
        # "#CSM \"Data: Initialize\"\nInitialize the shift-register data, here.\n(data names are defined by what you wire into the bundle function)"
        n51 = Bundle("Core"=w177, "Your Boolean data"=w179, "Your string data"=w178) -> (w181:T4)  [unwired: 1 in]
        n52 = call <vilib>:"Add State(s) to Queue__JKI_lib_State_Machine.vi"("State(s) in (\"\")"=w183) -> ("States Out"=w182:string)  [unwired: 14 in]
      }
      frame "Data: Cleanup" {
        # "#CSM \"Data: Cleanup\"\nCleanup any data and references, here.\n(this is called automatically, by the Macro: Exit)"
        n53 = Unbundle By Name(w185) -> ("Core.Current VI Reference"=w188:refnum<vi>)
        n54 = Close Reference(reference=w188, error in (no error)=w187) -> (error out=w186:errorcluster)
        n55 = call <vilib>:"Add State(s) to Queue__JKI_lib_State_Machine.vi"("State(s) in (\"\")"=w190) -> ("States Out"=w189:string)  [unwired: 14 in]
      }
      frame "---------- Events ----------" {
        # "#CSM \"Category Seperator\"\nDo not put any code in this frame."
        n56 = call <vilib>:"Add State(s) to Queue__JKI_lib_State_Machine.vi"("State(s) in (\"\")"=w195) -> ("States Out"=w194:string)  [unwired: 14 in]
      }
      frame "Events: Register" {
        # "#CSM \"Events: Register\"\nRegister user event. New Message Event is registered to break CSM waiting in event structure by default."
        # "#CSM Register New Message Event\nRegister message event to break Waiting in Event structure."
        n57 = call "CSM - Get New State Notifier Event.vi"("Name(\"\" to use uuid) in"=w199) -> ("Error out"=w197:errorcluster, "New State Notifier Event"=w198:refnum<user-event>)  [unwired: 9 in]
        n58 = register-events(error in=w197, w198) -> (reference out=w200:refnum<event-registration>, error out=w196:errorcluster)  [unwired: 1 in]
      }
      frame "Events: Unregister" {
        # "#CSM \"Events: Unregister\"\nUnregister user event."
        n59 = Unregister For Events(event registration refnum=w203, error in=w207) -> (error out=w204:errorcluster)
      }
      frame "---------- UI ----------" {
        # "#CSM \"Category Seperator\"\nDo not put any code in this frame."
        n60 = call <vilib>:"Add State(s) to Queue__JKI_lib_State_Machine.vi"("State(s) in (\"\")"=w212) -> ("States Out"=w211:string)  [unwired: 14 in]
      }
      frame "UI: Initialize" {
        # "#CSM \"UI: Initialize\"\nInitialize the User Interface, here.\n(this is called automatically, by the Macro: Init)"
        n61 = call <vilib>:"Add State(s) to Queue__JKI_lib_State_Machine.vi"("State(s) in (\"\")"=w217) -> ("States Out"=w216:string)  [unwired: 14 in]
      }
      frame "UI: Cursor Set" {
        # "Argument"
        # "#CSM \"UI: Cursor Set\"\nSet and Unset Cursor Busy.\n(Usage: \"UI: Cursor Set >> Busy|Idle\")"
        n62 = disable-structure shown="Default" {
          disable-tunnel: w221 -> [w227 w232]
          disable-tunnel: [w226 w232] -> w220
          disable-tunnel: w219 -> [w225 _]
          frame condition #0 (active) {
            n63 = case shown="\"Busy\"" w225 {
              tunnel: w227 -> [w229 w231]
              tunnel: [w228 w230] -> w226
              frame "Idle", Default {
                n64 = call <vilib>:"Unset Busy.vi"("error in (no error)"=w229) -> ("error out"=w228:errorcluster)  [unwired: 10 in]
              }
              frame "Busy" {
                n65 = call <vilib>:"Set Busy.vi"("error in (no error)"=w231) -> ("error out"=w230:errorcluster)  [unwired: 9 in, 1 out]
              }
            }
          }
          frame condition #1 {
          }
        }
        n66 = call <vilib>:"Add State(s) to Queue__JKI_lib_State_Machine.vi"("State(s) in (\"\")"=w224) -> ("States Out"=w223:string)  [unwired: 14 in]
      }
      frame "UI: Front Panel State" {
        # "Argument"
        # "#CSM \"UI: Front Panel State\"\nSet Front Panel Open or Closed\n(Usage: \"UI: Front Panel State >> Open|Close\")"
        n67 = Unbundle By Name(w236) -> ("Core.Current VI Reference"=w235:refnum<vi>)
        n68 = case shown="\"Minimize\", \"Minimized\"" w234 {
          tunnel: w238 -> [w246 w261 w272 w285 w298]
          tunnel: [w248 w262 w274 w287 w300] -> w237
          tunnel: w235 -> [w247 w259 w273 w286 w299]
          frame "Open", "Standard", Default {
            w241 = T1."Standard" ("State")
            n69 = property class="VI"(reference=w247, error in=w246) -> (reference out=w244:refnum<vi>, error out=w245:errorcluster, "FP.State"=w243:T1)
            n70 = Not Equal?(x=w243, y=w241) -> (x != y?=w242:bool)
            n71 = case shown="True" w242 {
              tunnel: [w252 w254] -> w248
              tunnel: w245 -> [w251 w254]
              tunnel: w244 -> [w250 _]
              tunnel: w241 -> [w249 _]
              frame True {
                n72 = invoke class="VI" method="FP.Open"(reference=w250, error in=w251, "Activate"=TRUE, "State"=w249) -> (error out=w252:errorcluster)  [unwired: 1 in, 4 out]
              }
              frame False {
              }
            }
          }
          frame "Close", "Closed" {
            n73 = property class="VI"(reference=w259, error in=w261) -> (reference out=w258:refnum<vi>, error out=w260:errorcluster, "FP.State"=w256:T1)
            n74 = Not Equal?(x=w256, y=T1."Closed" ("Front Panel Window:State")) -> (x != y?=w255:bool)
            n75 = case shown="True" w255 {
              tunnel: [w263 w266] -> w262
              tunnel: w260 -> [w263 w265]
              tunnel: w258 -> [_ w264]
              frame False {
              }
              frame True {
                n76 = invoke class="VI" method="FP.Close"(reference=w264, error in=w265) -> (error out=w266:errorcluster)  [unwired: 1 in, 2 out]
              }
            }
          }
          frame "Hidden", "Hide" {
            w267 = T1."Hidden" ("State")
            n77 = property class="VI"(reference=w273, error in=w272) -> (reference out=w270:refnum<vi>, error out=w271:errorcluster, "FP.State"=w269:T1)
            n78 = Not Equal?(x=w269, y=w267) -> (x != y?=w268:bool)
            n79 = case shown="True" w268 {
              tunnel: [w278 w279] -> w274
              tunnel: w271 -> [w277 w279]
              tunnel: w270 -> [w276 _]
              tunnel: w267 -> [w275 _]
              frame True {
                n80 = invoke class="VI" method="FP.Open"(reference=w276, error in=w277, "State"=w275) -> (error out=w278:errorcluster)  [unwired: 2 in, 4 out]
              }
              frame False {
              }
            }
          }
          frame "Minimize", "Minimized" {
            w280 = T1."Minimized" ("State")
            n81 = property class="VI"(reference=w286, error in=w285) -> (reference out=w283:refnum<vi>, error out=w284:errorcluster, "FP.State"=w282:T1)
            n82 = Not Equal?(x=w282, y=w280) -> (x != y?=w281:bool)
            n83 = case shown="False" w281 {
              tunnel: [w291 w292] -> w287
              tunnel: w284 -> [w290 w292]
              tunnel: w283 -> [w289 _]
              tunnel: w280 -> [w288 _]
              frame True {
                n84 = invoke class="VI" method="FP.Open"(reference=w289, error in=w290, "State"=w288) -> (error out=w291:errorcluster)  [unwired: 2 in, 4 out]
              }
              frame False {
              }
            }
          }
          frame "Maximize", "Maximized" {
            w293 = T1."Maximized" ("State")
            n85 = property class="VI"(reference=w299, error in=w298) -> (reference out=w296:refnum<vi>, error out=w297:errorcluster, "FP.State"=w295:T1)
            n86 = Not Equal?(x=w295, y=w293) -> (x != y?=w294:bool)
            n87 = case shown="True" w294 {
              tunnel: [w304 w305] -> w300
              tunnel: w297 -> [w303 w305]
              tunnel: w296 -> [w302 _]
              tunnel: w293 -> [w301 _]
              frame True {
                n88 = invoke class="VI" method="FP.Open"(reference=w302, error in=w303, "State"=w301) -> (error out=w304:errorcluster)  [unwired: 2 in, 4 out]
              }
              frame False {
              }
            }
          }
        }
        n89 = call <vilib>:"Add State(s) to Queue__JKI_lib_State_Machine.vi"("State(s) in (\"\")"=w240) -> ("States Out"=w239:string)  [unwired: 14 in]
      }
      frame "---------- Macro ----------" {
        # "#CSM \"Category Seperator\"\nDo not put any code in this frame."
        n90 = call <vilib>:"Add State(s) to Queue__JKI_lib_State_Machine.vi"("State(s) in (\"\")"=w310) -> ("States Out"=w309:string)  [unwired: 14 in]
      }
      frame "Macro: Initialize" {
        w312 = "Data: Initialize\nInitialize Core Data\nEvents: Register\nUI: Initialize\nUI: Front Panel State >> Open"  # Data: Initialize Initialize Core Data Events: Register UI: Initialize UI: Front Panel State >> Open
        # "#CSM \"Macro: Initialize\"\nInitialization Macro (This is called once, when the VI starts)"
        n91 = call <vilib>:"Add State(s) to Queue__JKI_lib_State_Machine.vi"("State(s) in Front (\"\")"=w312, "State(s) in (\"\")"=w316) -> ("States Out"=w315:string)  [unwired: 13 in]
      }
      frame "Macro: Exit" {
        # "#CSM \"Macro: Exit\"\nExit Macro (This is called once, when the VI exits)"
        n92 = Unbundle By Name(w325) -> ("Core.Close Panel on Exit?"=w324:bool)
        n93 = Select(t="UI: Front Panel State >> Close", s=w324, f="") -> (s? t:f=w321:string)
        n94 = call <vilib>:"Add State(s) to Queue__JKI_lib_State_Machine.vi"("State(s) in Front (\"\")"="//Exit Sub-Modules ", "State(s) in (\"\")"=w321, "State(s) at Back (\"\")"="Data: Cleanup\nEvents: Unregister\nExit") -> ("States Out"=w319:string)  [unwired: 12 in]
        n95 = call <vilib>:"Add State(s) to Queue__JKI_lib_State_Machine.vi"("State(s) in Front (\"\")"=w319, "State(s) in (\"\")"=w328) -> ("States Out"=w327:string)  [unwired: 13 in]
      }
      frame "---------- API ----------" {
        # "#CSM \"Category Seperator\"\nDo not put any code in this frame."
      }
      frame "API: API1" {
        # "#CSM >> Source CSM >>\nIf you need to tell who triggered this state , use this string. If it's this case itself, this string is \"\"."
        # "#CSM >> Arguments >>\nDeal with the parameter if any"
        # "#CSM Response\nConnect this to return the response of your API"
        # "#CSM API Example\nCopy/Rename this case for your own API"
      }
      frame "API: API2" {
        # "#CSM API Example\nCopy/Rename this case for your own API"
      }
      frame "---------- DoSth ----------" {
        # "#CSM \"Category Seperator\"\nDo not put any code in this frame."
        n96 = call <vilib>:"Add State(s) to Queue__JKI_lib_State_Machine.vi"("State(s) in (\"\")"=w346) -> ("States Out"=w345:string)  [unwired: 14 in]
      }
      frame "DoSth: DoA" {
        # "#CSM \"Internal State\"\nThis category is used for holding internal states"
        n97 = call <vilib>:"Add State(s) to Queue__JKI_lib_State_Machine.vi"("State(s) in (\"\")"=w351) -> ("States Out"=w350:string)  [unwired: 14 in]
      }
      frame "DoSth: DoB" {
        # "#CSM \"Internal State\"\nThis category is used for holding internal states"
        n98 = call <vilib>:"Add State(s) to Queue__JKI_lib_State_Machine.vi"("State(s) in (\"\")"=w356) -> ("States Out"=w355:string)  [unwired: 14 in]
      }
    }
  }
